vi "Read OptiTrack Config.vi"() -> (0 "error out":errorcluster, 3 "Offset Array":dbl[](array[numeric]) format="%.4f")   [LabVIEW 2022 SP3]
uses:
  Anemometry/Anemometry Sub Vis/Globals/Constants_global.vi
  <vilib>/Utility/config.llb/Read Key (String).vi
  <vilib>/Utility/config.llb/NI_LVConfig.lvlib
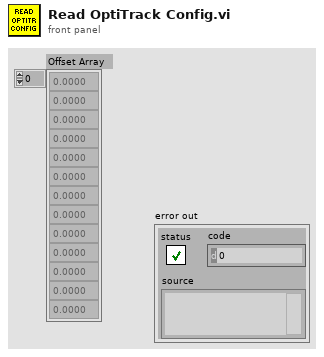
[diagram p1: front panel]
types:
  T1 = typedef "NI_LVConfig.lvlib/Config Data RefNum.ctl" = refnum<k1>
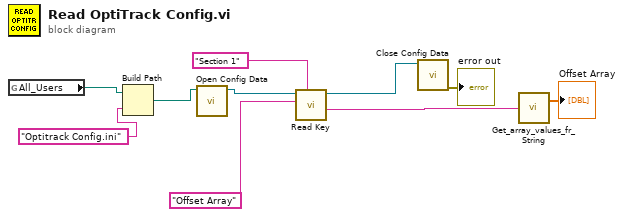
[diagram p0: block diagram]
diagram:
  n1 = global read "Constants_global.vi" "All_Users"() -> (w10:path)
  n2 = Build Path(base path=w10, name or relative path="Optitrack Config.ini") -> (appended path=w8:path)
  n3 = call <vilib>:"Open Config Data.vi"("configuration file path"=w8) -> ("refnum"=w5:T1)  [unwired: 2 in, 8 out]
  n4 = call-poly <vilib>:"Read Key.vi"("section"="Section 1", "key"="Offset Array", "refnum"=w5) -> ("value"=w4:string, "refnum out"=w2:T1)  [unwired: 5 in, 2 out]
  n5 = call <vilib>:"Close Config Data.vi"("refnum"=w2) -> ("error out"=→"error out":errorcluster)  [unwired: 9 in, 1 out]
  n6 = call "Get_array_values_fr_String.vi"("String Value"=w4) -> ("Numeric Array"=→"Offset Array":dbl[])  [unwired: 1 out]
